vi "Delete Source Module.vi"(0 "BroadcastRegistry in":refnum<class "BroadcastRegistry.lvclass">, 7 "Source":string) -> (4 "BroadcastRegistry out":refnum<class "BroadcastRegistry.lvclass">)   [LabVIEW 2020, in "Communicable State Machine.lvlib" / "BroadcastRegistry.lvclass"]
uses:
  BroadcastRegistry.lvclass
  BroadcastRegistry.lvclass/BroadcastRegistry.ctl
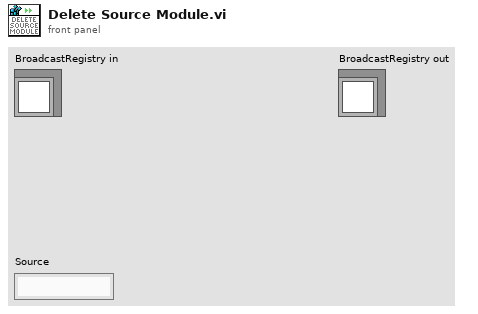
[diagram p1: front panel]
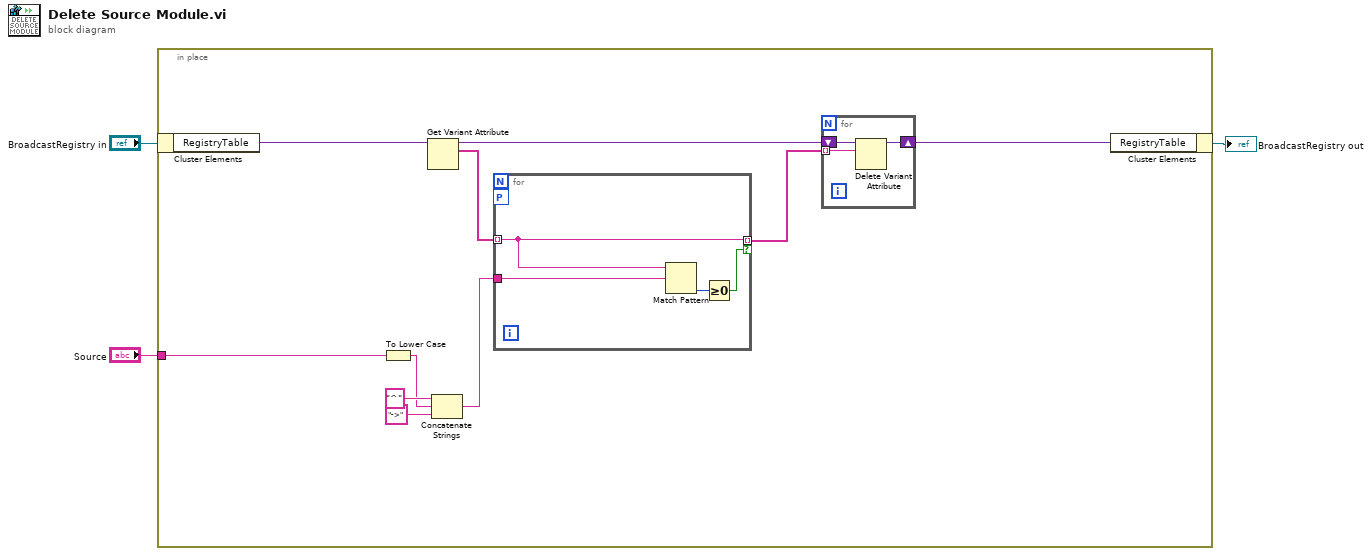
[diagram p0: block diagram]
diagram:
  n1 = in-place {
    in-place-border: "Source" -> [w4]
    n2 = in-place-cluster #1("BroadcastRegistry in") -> ("RegistryTable"=w13:variant)
    n3 = To Lower Case(string=w4) -> (all lower case string=w6:string)
    n4 = Get Variant Attribute(Variant=w13) -> (duplicate Variant=w11:variant, names=w10:string[])  [unwired: 3 in, 2 out]
    n5 = Concatenate Strings("^" ("string"), w6, "->" ("string")) -> (w7:string)
    n6 = for {
      tunnel: w10 -> [w20] mode=indexing
      tunnel: [w20] -> w9 mode=indexing if=w17
      tunnel: w7 -> [w19]
      workers-P: _ -> [_]
      n7 = Match Pattern(string=w20, regular expression=w19) -> (offset past match=w18:i32)  [unwired: 1 in, 3 out]
      n8 = Greater Or Equal To 0?(x=w18) -> (x >= 0?=w17:bool)
    }
    n9 = for {
      tunnel: w9 -> [w14] mode=indexing
      shift-right: [w16] -> w5
      shift-left: w11 -> [w15]
      n10 = Delete Variant Attribute(6:w14, 7:w15) -> (3:w16:variant)  [unwired: 1 in, 2 out]
    }
    n11 = in-place-cluster #1("RegistryTable"=w5) -> (→"BroadcastRegistry out":refnum<class "BroadcastRegistry.lvclass">)
  }
